vi "Configure Trigger (Communication).vi"(0 "VISA resource name":refnum<visa-resource-name>, 1 "Encoding Type (0: RZ)":i32(ring) items=["RZ", "NRZ"], 5 "Trigger Source (1: Channel1)":i32(ring)=1 items=["Channel1"=1, "Channel2"=2, "Channel3"=3, "Channel4"=4], 7 "Bit Width (1E-7 s)":dbl=1e-07, 9 "Trigger Polarity (0: Negative)":i32(ring) items=["Negative", "Positive"], 11 "error in (no error)":errorcluster, 12 "Trigger Pattern":i32[](array[ring])=[1, 0, 1] items=["-1"=-1, "1"=1, "0"=0]) -> (4 "VISA resource name out":refnum<visa-resource-name>, 15 "error out":errorcluster)   [LabVIEW 2013, in "Agilent 90000 Series.lvlib"]
doc: "Configures the communication trigger parameters."
uses:
  Agilent 90000 Series.lvlib
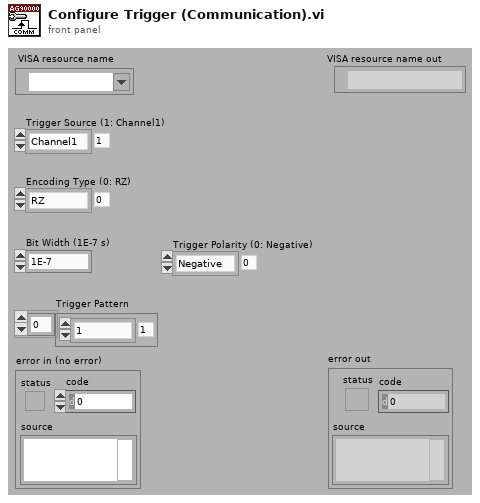
[diagram p1: front panel]
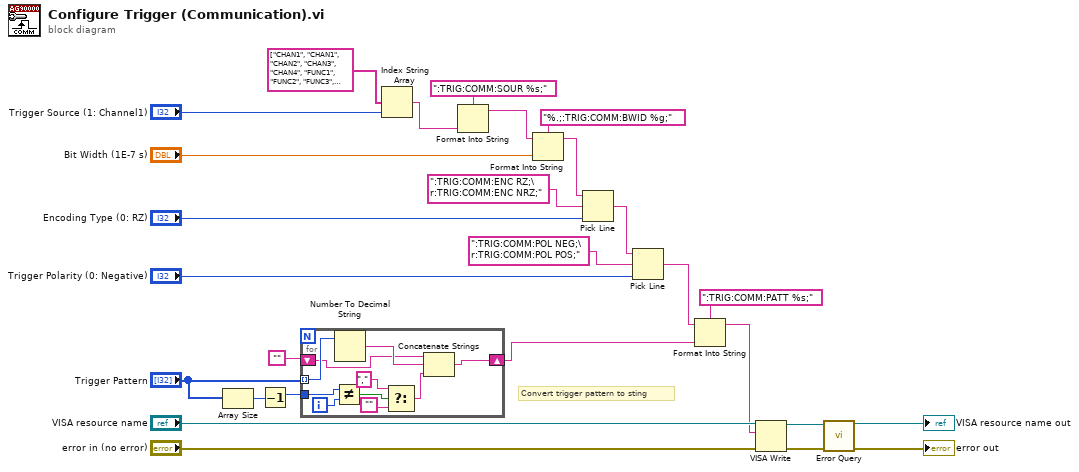
[diagram p0: block diagram]
diagram:
  # "Convert trigger pattern to sting"
  n1 = Array Size(array="Trigger Pattern") -> (size(s)=w6:i32)
  n2 = Decrement(x=w6) -> (x-1=w5:i32)
  n3 = for {
    tunnel: "Trigger Pattern" -> [w37] mode=indexing
    shift-right: [w35] -> w3
    shift-left: "" -> [w34]
    tunnel: w5 -> [w33]
    i -> [w32]
    n4 = Not Equal?(x=w33, y=w32) -> (x != y?=w31:bool)
    n5 = Number To Decimal String(number=w37) -> (decimal integer string=w36:string)  [unwired: 1 out]
    n6 = Select(t="," ("string"), s=w31, f="") -> (s? t:f=w28:string)
    n7 = Concatenate Strings(w34, w36, w28) -> (w35:string)
  }
  n8 = Index String Array(1:"Trigger Source (1: Channel1)", 2:string[] ["CHAN1", "CHAN1", "CHAN2", "CHAN3", "CHAN4", "FUNC1", "FUNC2", "FUNC3", "FUNC4", "WMEM1", "WMEM2", "WMEM3", "WMEM4", "AUX", "LINE"]) -> (0:w9:string)  [unwired: 1 out]
  n9 = Format Into String(format string=":TRIG:COMM:SOUR %s;", w9) -> (resulting string=w26:string)  [unwired: 2 in, 1 out]
  n10 = Format Into String(format string="%.;:TRIG:COMM:BWID %g;", initial string=w26, "Bit Width (1E-7 s)") -> (resulting string=w23:string)  [unwired: 1 in, 1 out]
  n11 = Pick Line(string ("")=w23, multi-line string=":TRIG:COMM:ENC RZ;\r:TRIG:COMM:ENC NRZ;", line index="Encoding Type (0: RZ)") -> (output string=w20:string)
  n12 = Pick Line(string ("")=w20, multi-line string=":TRIG:COMM:POL NEG;\r:TRIG:COMM:POL POS;", line index="Trigger Polarity (0: Negative)") -> (output string=w4:string)
  n13 = Format Into String(format string=":TRIG:COMM:PATT %s;", initial string=w4, w3) -> (resulting string=w1:string)  [unwired: 1 in, 1 out]
  n14 = VISA Write(VISA resource name="VISA resource name", write buffer=w1, error in (no error)="error in (no error)") -> (VISA resource name out=w15:refnum<visa-resource-name>, error out=w14:errorcluster)  [unwired: 1 out]
  n15 = call "Error Query.vi"("error in (no error)"=w14, "VISA resource name"=w15) -> ("error out"=→"error out":errorcluster, "VISA resource name out"=→"VISA resource name out":refnum<visa-resource-name>)  [unwired: 8 out]
